vi "StartVeriStandBundle_Create Reference Locals.vi"(5 "Sequence Context":refnum<k7>) -> (0 "error out":errorcluster)   [LabVIEW 2015, in "MiscHelperVIs.lvlib"]
uses:
  MiscHelperVIs.lvlib
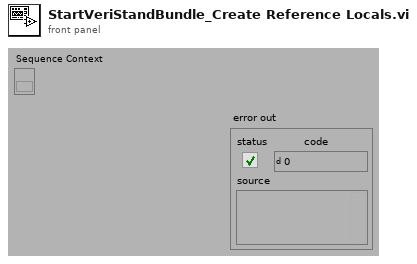
[diagram p1: front panel]
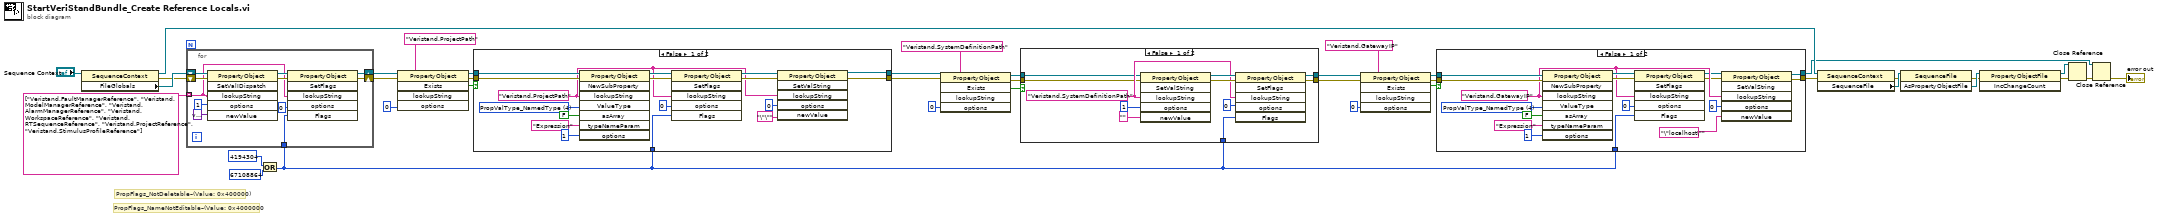
[diagram p0: block diagram]
diagram:
  # "PropFlags_NotDeletable–(Value: 0x400000)"
  # "PropFlags_NameNotEditable–(Value: 0x4000000"
  n1 = property class="SequenceContext"(reference="Sequence Context") -> (reference out=w37:refnum<k7>, error out=w28:errorcluster, "FileGlobals"=w39:refnum<k7>)  [unwired: 1 in]
  n2 = Or(x=4194304 ("Flags"), y=67108864 ("Flags")) -> (x .or. y?=w21:i32)
  n3 = for {
    shift-right: [w44] -> w27
    shift-left: w39 -> [w50]
    tunnel: string[] ["Veristand.FaultManagerReference", "Veristand.ModelManagerReference", "Veristand.AlarmManagerReference", "Veristand.WorkspaceReference", "Veristand.RTSequenceReference", "Veristand.ProjectReference", "Veristand.StimulusProfileReference"] -> [w40] mode=indexing
    shift-right: [w43] -> w26
    shift-left: w28 -> [w47]
    tunnel: w21 -> [w42]
    n4 = invoke class="PropertyObject" method="SetValIDispatch"(reference=w50, error in=w47, "lookupString"=w40, "options"=1, "newValue"=variant) -> (reference out=w46:refnum<k7>, error out=w45:errorcluster)  [unwired: 1 in, 4 out]
    n5 = invoke class="PropertyObject" method="SetFlags"(reference=w46, error in=w45, "lookupString"=w40, "options"=0, "Flags"=w42) -> (reference out=w44:refnum<k7>, error out=w43:errorcluster)  [unwired: 1 in, 4 out]
  }
  n6 = invoke class="PropertyObject" method="Exists"(reference=w27, error in=w26, "lookupString"="Veristand.ProjectPath", "options"=0) -> (reference out=w3:refnum<k7>, error out=w4:errorcluster, "Exists"=w2:bool)  [unwired: 1 in, 2 out]
  n7 = case shown="False" w2 {
    tunnel: w3 -> [w67 w69]
    tunnel: w4 -> [w66 w68]
    tunnel: [w52 w68] -> w17
    tunnel: [w51 w69] -> w18
    tunnel: w21 -> [w59 _]
    frame False {
      w64 = 4 items=["PropValType_Container", "PropValType_String", "PropValType_Boolean", "PropValType_Number", "PropValType_NamedType", "PropValType_Reference", "PropValType_Array"] ("ValueType")
      w55 = "Veristand.ProjectPath"
      n8 = invoke class="PropertyObject" method="NewSubProperty"(reference=w67, error in=w66, "lookupString"=w55, "ValueType"=w64, "asArray"=FALSE, "typeNameParam"="Expression", "options"=1) -> (reference out=w61:refnum<k7>, error out=w60:errorcluster)  [unwired: 1 in, 6 out]
      n9 = invoke class="PropertyObject" method="SetFlags"(reference=w61, error in=w60, "lookupString"=w55, "options"=0, "Flags"=w59) -> (reference out=w57:refnum<k7>, error out=w56:errorcluster)  [unwired: 1 in, 4 out]
      n10 = invoke class="PropertyObject" method="SetValString"(reference=w57, error in=w56, "lookupString"=w55, "options"=0, "newValue"="\"\"") -> (reference out=w51:refnum<k7>, error out=w52:errorcluster)  [unwired: 1 in, 4 out]
    }
    frame True {
    }
  }
  n11 = invoke class="PropertyObject" method="Exists"(reference=w18, error in=w17, "lookupString"="Veristand.SystemDefinitionPath", "options"=0) -> (reference out=w8:refnum<k7>, error out=w7:errorcluster, "Exists"=w9:bool)  [unwired: 1 in, 2 out]
  n12 = case shown="False" w9 {
    tunnel: w21 -> [w74 _]
    tunnel: [w73 w81] -> w20
    tunnel: [w72 w82] -> w19
    tunnel: w8 -> [w71 w82]
    tunnel: w7 -> [w70 w81]
    frame False {
      w75 = "Veristand.SystemDefinitionPath"
      n13 = invoke class="PropertyObject" method="SetValString"(reference=w71, error in=w70, "lookupString"=w75, "options"=1, "newValue"="") -> (reference out=w77:refnum<k7>, error out=w76:errorcluster)  [unwired: 1 in, 4 out]
      n14 = invoke class="PropertyObject" method="SetFlags"(reference=w77, error in=w76, "lookupString"=w75, "options"=0, "Flags"=w74) -> (reference out=w72:refnum<k7>, error out=w73:errorcluster)  [unwired: 1 in, 4 out]
    }
    frame True {
    }
  }
  n15 = invoke class="PropertyObject" method="Exists"(reference=w19, error in=w20, "lookupString"="Veristand.GatewayIP", "options"=0) -> (reference out=w15:refnum<k7>, error out=w14:errorcluster, "Exists"=w16:bool)  [unwired: 1 in, 2 out]
  n16 = case shown="False" w16 {
    tunnel: w15 -> [w99 w101]
    tunnel: w14 -> [w98 w100]
    tunnel: [w84 w100] -> w22
    tunnel: [w83 w101] -> w23
    tunnel: w21 -> [w91 _]
    frame False {
      w96 = 4 items=["PropValType_Container", "PropValType_String", "PropValType_Boolean", "PropValType_Number", "PropValType_NamedType", "PropValType_Reference", "PropValType_Array"] ("ValueType")
      w87 = "Veristand.GatewayIP"
      n17 = invoke class="PropertyObject" method="NewSubProperty"(reference=w99, error in=w98, "lookupString"=w87, "ValueType"=w96, "asArray"=FALSE, "typeNameParam"="Expression", "options"=1) -> (reference out=w93:refnum<k7>, error out=w92:errorcluster)  [unwired: 1 in, 6 out]
      n18 = invoke class="PropertyObject" method="SetFlags"(reference=w93, error in=w92, "lookupString"=w87, "options"=0, "Flags"=w91) -> (reference out=w86:refnum<k7>, error out=w85:errorcluster)  [unwired: 1 in, 4 out]
      n19 = invoke class="PropertyObject" method="SetValString"(reference=w86, error in=w85, "lookupString"=w87, "options"=0, "newValue"="\"localhost\"") -> (reference out=w83:refnum<k7>, error out=w84:errorcluster)  [unwired: 1 in, 4 out]
    }
    frame True {
    }
  }
  n20 = property class="SequenceContext"(reference=w37, error in=w22) -> (error out=w35:errorcluster, "SequenceFile"=w36:refnum<k7>)  [unwired: 1 out]
  n21 = invoke class="SequenceFile" method="AsPropertyObjectFile"(reference=w36, error in=w35) -> (error out=w33:errorcluster, "AsPropertyObjectFile"=w34:refnum<k7>)  [unwired: 1 in, 1 out]
  n22 = invoke class="PropertyObjectFile" method="IncChangeCount"(reference=w34, error in=w33) -> (reference out=w31:refnum<k7>, error out=w32:errorcluster)  [unwired: 1 in, 1 out]
  n23 = Close Reference(reference=w31, error in (no error)=w32) -> (error out=w30:errorcluster)
  n24 = Close Reference(reference=w23, error in (no error)=w30) -> (error out=→"error out":errorcluster)
